vi "please delete path finder test.vi"() -> ()   [LabVIEW 2015]
panel:
  out "path":path
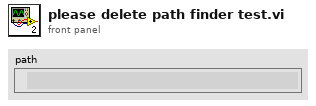
[diagram p1: front panel]
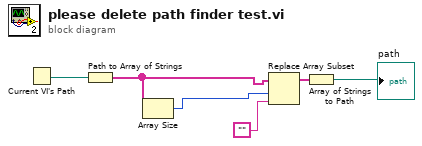
[diagram p0: block diagram]
diagram:
  n1 = Current VI's Path() -> (path=w6:path)
  n2 = Path to Array of Strings(0:w6) -> (2:w3:string[])  [unwired: 1 out]
  n3 = Array Size(array=w3) -> (size(s)=w2:i32)
  n4 = Replace Array Subset(array=w3, new element="", index=w2) -> (w1:string[])
  n5 = Array of Strings to Path(0:w1) -> (2:→"path":path)  [unwired: 1 in]
